vi "SL9200 Volume Test.vi"() -> ()   [LabVIEW 2009]
uses:
  SL9200_Registers.ctl
panel:
  in  "Starting Offset":dbl
  out "Riter Reading":dbl format="%#_8g"
  in  "stop 2":bool
  out "Error Out":errorcluster
  out "V(0)":dbl
  in  "ComPort":refnum<visa-resource-name>="COM1"
  out "Numeric":i32
  in  "Start":bool
  in  "Init Dial":sgl(knob) scale=0.0..3.0
  out "Riter Dial":sgl(knob) scale=0.0..3.0
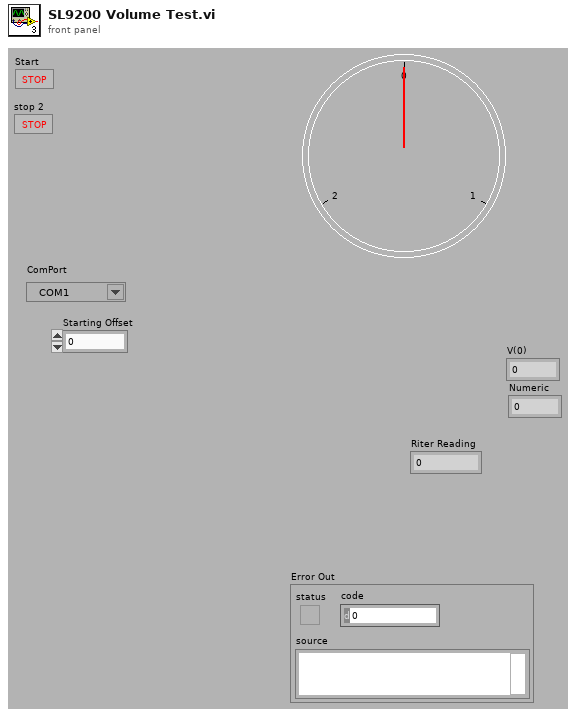
[diagram p1: front panel]
types:
  T1 = typedef "SL9200_Registers.ctl" = u8
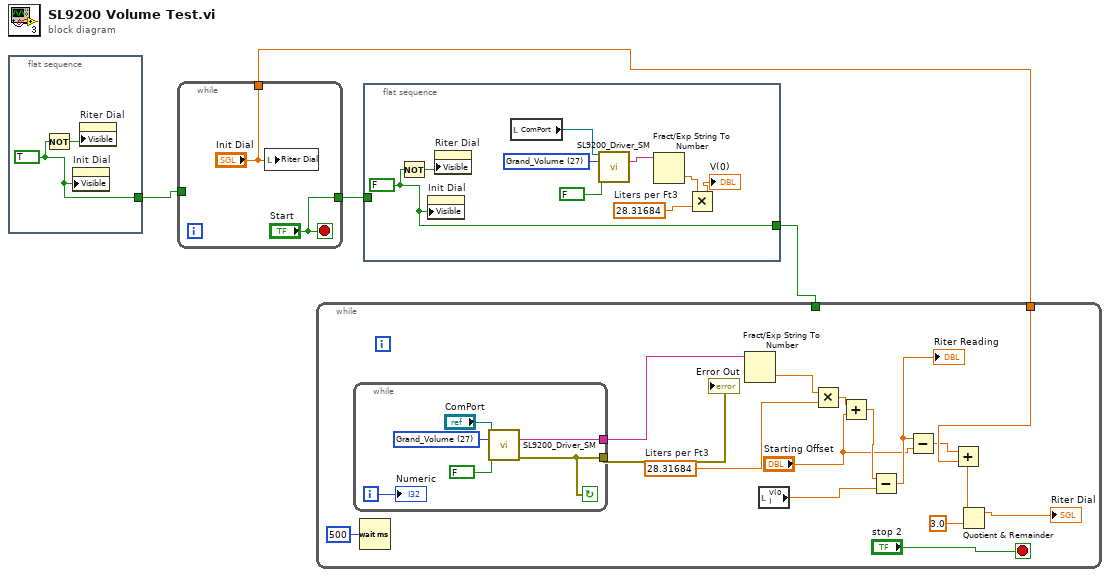
[diagram p0: block diagram]
diagram:
  n1 = flat-sequence {
    tunnel: [w5] -> w4
    frame #0 {
      w5 = TRUE ("Visible")
      n2 = Not(x=w5) -> (.not. x?=w6:bool)
      n3 = property on="Init Dial" class="Knob (strict)"("Visible"=w5) -> ()  [unwired: 2 in, 2 out]
      n4 = property on="Riter Dial" class="Knob (strict)"("Visible"=w6) -> ()  [unwired: 2 in, 2 out]
    }
  }
  n5 = while {
    tunnel: ["Init Dial"] -> w2
    tunnel: w4 -> [_]
    tunnel: ["Start"] -> w3
    stop <- "Start" stop-if-true
    n6 = local write "Riter Dial"("Init Dial") -> ()
  }
  n7 = while {
    tunnel: w2 -> [w12]
    tunnel: w1 -> [_]
    stop <- "stop 2" stop-if-true
    w23 = 28.31684  # Liters per Ft3
    n8 = while {
      tunnel: [w28] -> w24
      tunnel: [w26] -> w20
      i -> [w25]
      stop <- w26 continue-if-true
      w30 = T1 27 items=["Heat_Flow", "Mass_Flow", "Corrected_Volume_Flow", "Volume_Flow", "Temperature", "Temperature2", "Delta_Temperature", "Pressure", "Diff_Pressure", "Density", "Spec_Enthalpy", "Date", "Time", "Level", "Peak_Demand", "Demand_Last_Hour", "Peak_Demand_Time", "Peak_Demand_Date", "Viscosity", "Reynolds_Number", "Heat_Total", "Grand_Heat_Total", "Mass_Total", "Grand_Mass", "Corrected_Volume_Total", "Grand_Corrected_Volume", "Volume_Total", "Grand_Volume", "Totalizer_Reset", "Alarm_Reset", "Barometric", "Fluid_Type", "Reference_Density", "Therm_Expansion_Coef", "Combustion_Heat", "Specific_Heat", "Flow_Z_Factor", "Ref_Z_Factor", "Isentropic_Exponent", "Viscosity_A", "Viscosity_B", "Reference_Temperature", "Calibration_Density", "Base_Density_H2O_4C", "Per_Mole_N2", "Per_Mole_CO2", "Tag_Number", "Software_Version", "Hardware_Version", "Order_Code", "Serial_Number", "Sensor_Serial_Num"] ("Register")
      n9 = call "SL9200_Driver_SM.vi"("ComPort"="ComPort", "Register"=w30, "InitSerial?"=FALSE) -> ("Response"=w28:string, "Error Out"=w26:errorcluster)  [unwired: 10 in, 1 out]
      "Numeric" <- w25
    }
    "Error Out" <- w20
    n10 = Wait (ms)(milliseconds to wait=u32 500) -> ()  [unwired: 1 out]
    n11 = Fract/Exp String To Number(string=w24) -> (number=w15:dbl)  [unwired: 3 in, 1 out]
    n12 = local read "V(0)"() -> (w13:dbl)
    n13 = Multiply(x=w15, y=w23) -> (x*y=w22:dbl)
    n14 = Add(x=w22, y="Starting Offset") -> (x+y=w14:dbl)
    n15 = Subtract(x=w14, y=w13) -> (x-y=w10:dbl)
    "Riter Reading" <- w10
    n16 = Subtract(x=w10, y="Starting Offset") -> (x-y=w11:dbl)
    n17 = Add(x=w11, y=w12) -> (x+y=w18:dbl)
    n18 = Quotient & Remainder(x=w18, y=3.0) -> (x-y*floor(x/y)=→"Riter Dial":dbl)  [unwired: 1 out]
  }
  n19 = flat-sequence {
    tunnel: [w38] -> w1
    tunnel: w3 -> [_]
    frame #0 {
      w33 = 28.31684  # Liters per Ft3
      w36 = T1 27 items=["Heat_Flow", "Mass_Flow", "Corrected_Volume_Flow", "Volume_Flow", "Temperature", "Temperature2", "Delta_Temperature", "Pressure", "Diff_Pressure", "Density", "Spec_Enthalpy", "Date", "Time", "Level", "Peak_Demand", "Demand_Last_Hour", "Peak_Demand_Time", "Peak_Demand_Date", "Viscosity", "Reynolds_Number", "Heat_Total", "Grand_Heat_Total", "Mass_Total", "Grand_Mass", "Corrected_Volume_Total", "Grand_Corrected_Volume", "Volume_Total", "Grand_Volume", "Totalizer_Reset", "Alarm_Reset", "Barometric", "Fluid_Type", "Reference_Density", "Therm_Expansion_Coef", "Combustion_Heat", "Specific_Heat", "Flow_Z_Factor", "Ref_Z_Factor", "Isentropic_Exponent", "Viscosity_A", "Viscosity_B", "Reference_Temperature", "Calibration_Density", "Base_Density_H2O_4C", "Per_Mole_N2", "Per_Mole_CO2", "Tag_Number", "Software_Version", "Hardware_Version", "Order_Code", "Serial_Number", "Sensor_Serial_Num"] ("Register")
      w38 = FALSE ("Visible")
      n20 = Not(x=w38) -> (.not. x?=w39:bool)
      n21 = property on="Init Dial" class="Knob (strict)"("Visible"=w38) -> ()  [unwired: 2 in, 2 out]
      n22 = property on="Riter Dial" class="Knob (strict)"("Visible"=w39) -> ()  [unwired: 2 in, 2 out]
      n23 = local read "ComPort"() -> (w35:refnum<visa-resource-name>)
      n24 = call "SL9200_Driver_SM.vi"("ComPort"=w35, "Register"=w36, "InitSerial?"=FALSE) -> ("Response"=w34:string)  [unwired: 10 in, 2 out]
      n25 = Fract/Exp String To Number(string=w34) -> (number=w32:dbl)  [unwired: 3 in, 1 out]
      n26 = Multiply(x=w32, y=w33) -> (x*y=→"V(0)":dbl)
    }
  }
